vi "Fire User Event - Stop.vi"(8 "error in (no error)":errorcluster, 9 "Event Data":variant, 10 "User Event":string, 11 "User Event in":refnum<user-event>) -> (0 "error out":errorcluster)   [LabVIEW 2019, in "User Event - Stop.lvlib"]
uses:
  All User Events.ctl
  User Event - Stop.lvlib
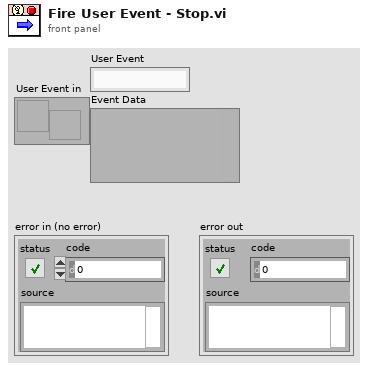
[diagram p1: front panel]
types:
  T1 = typedef "All User Events.ctl" = cluster{"User Event":string, "Event Data":variant}
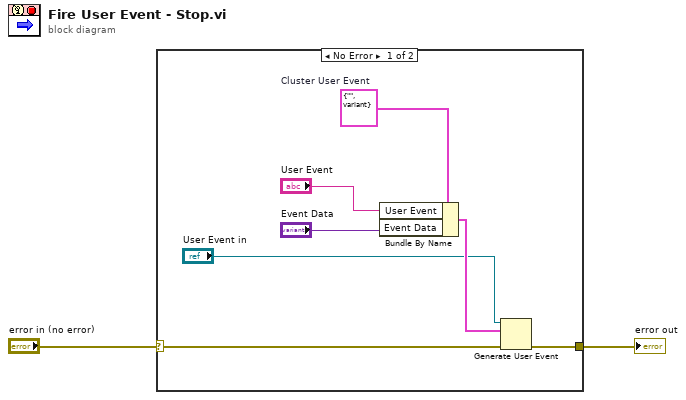
[diagram p0: block diagram]
diagram:
  n1 = case shown="No Error" "error in (no error)" {
    selector: "error in (no error)" -> [w3 w10]
    tunnel: [w6 w10] -> w2
    frame No Error {
      w8 = T1 {"User Event"="", "Event Data"=variant}  # Cluster User Event
      n2 = Bundle By Name(cluster=w8, "User Event"="User Event", "Event Data"="Event Data") -> (w9:T1)
      n3 = Generate User Event(user event="User Event in", event data cluster=w9, error in=w3) -> (error out=w6:errorcluster)  [unwired: 1 in, 1 out]
    }
    frame Error {
    }
  }
  "error out" <- w2
